vi "svl_Build dB Label (channel info).vi"(4 "width (-)":i16, 5 "number format":i16(ring) items=["Engineering", "Exponential", "Fractional", "Automatic"], 6 "include reference (T)":bool=TRUE, 7 "peak units":string, 8 "error in (no error)":errorcluster, 9 "precision (1)":i16=1, 10 "channel info":T1={"sensor sensitivity"=1000.0, "engineering units"=1, "dB reference"=1.0, "custom label"="EU", "weighting filter"=0, "pregain"=0.0} {"pregain" format="%.2f"; "weighting filter" items=["Linear", "A-weighting", "B-weighting", "C-weighting", "ITU-R 468-4", "Dolby", "CCITT", "C-message", "Wb", "Wc", "Wd", "We", "Wf", "Wh", "Wj", "Wk", "Wm", "AES17 20 kHz lowpass", "AES17 40 kHz lowpass", "AES17 20 kHz highpass", "AES17 40 kHz highpass"]; "dB reference" format="%^.1e"; "engineering units" items=["custom..."=0, "V"=1, "A"=21, "C"=30, "pC"=31, "s"=32, "-"=29, "Pa"=2, "N"=20, "g"=3, "m/s^2"=4, "m/s"=5, "m"=6, "mm/s"=12, "mm"=13, "micron/s"=14, "micron"=15, "in/s^2"=7, "in/s"=8, "in"=9, "mil/s"=10, "mil"=11, "rad/s^2"=16, "rad/s"=17, "rad"=18, "deg/s^2"=26, "deg/s"=27, "deg"=28, "RPM"=22, "cycle/s^2"=23, "Hz"=24, "cycle"=25, "strain"=19]; "sensor sensitivity" format="%#_5f"}, 11 "EU label":string) -> (0 "error out":errorcluster, 1 "dB reference [EU]":dbl format="%.2f", 2 "channel info":T1={"sensor sensitivity"=1000.0, "engineering units"=1, "dB reference"=1.0, "custom label"="EU", "weighting filter"=0, "pregain"=0.0} {"pregain" format="%.2f"; "weighting filter" items=["Linear", "A-weighting", "B-weighting", "C-weighting", "ITU-R 468-4", "Dolby", "CCITT", "C-message", "Wb", "Wc", "Wd", "We", "Wf", "Wh", "Wj", "Wk", "Wm", "AES17 20 kHz lowpass", "AES17 40 kHz lowpass", "AES17 20 kHz highpass", "AES17 40 kHz highpass"]; "dB reference" format="%^.1e"; "engineering units" items=["custom..."=0, "V"=1, "A"=21, "C"=30, "pC"=31, "s"=32, "-"=29, "Pa"=2, "N"=20, "g"=3, "m/s^2"=4, "m/s"=5, "m"=6, "mm/s"=12, "mm"=13, "micron/s"=14, "micron"=15, "in/s^2"=7, "in/s"=8, "in"=9, "mil/s"=10, "mil"=11, "rad/s^2"=16, "rad/s"=17, "rad"=18, "deg/s^2"=26, "deg/s"=27, "deg"=28, "RPM"=22, "cycle/s^2"=23, "Hz"=24, "cycle"=25, "strain"=19]; "sensor sensitivity" format="%#_5f"}, 3 "dB label":string)   [LabVIEW 2017]
uses:
  <vilib>/addons/_NISVFA/_Shared subVIs/Controls/svc_Channel Info.ctl
  <vilib>/addons/_NISVFA/_Shared subVIs/Controls/svc_Engineering Units Text Ring.ctl
  <vilib>/addons/_NISVFA/_Shared subVIs/Controls/svc_Weighting Filter Text Ring.ctl
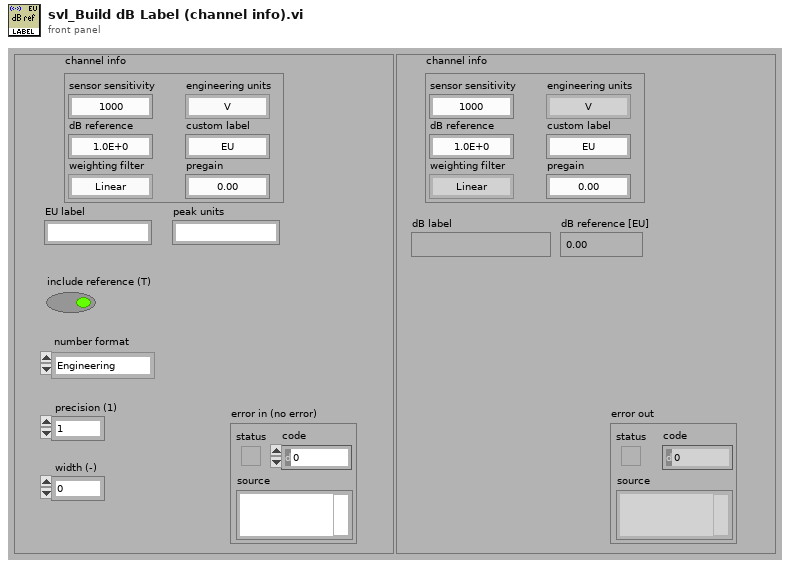
[diagram p1: front panel]
types:
  T1 = typedef "svc_Channel Info.ctl" = cluster{"sensor sensitivity":dbl, "engineering units":T2, "dB reference":dbl, "custom label":string, "weighting filter":T3, "pregain":dbl}
  T2 = typedef "svc_Engineering Units Text Ring.ctl" = u16
  T3 = typedef "svc_Weighting Filter Text Ring.ctl" = u16
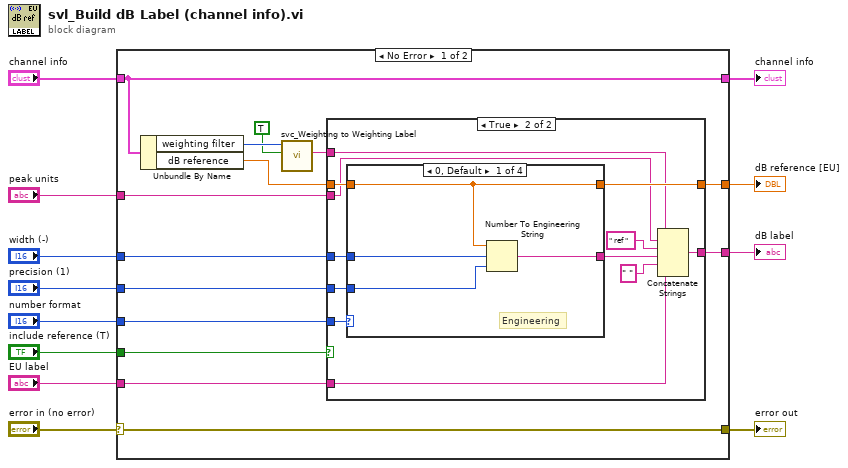
[diagram p0: block diagram]
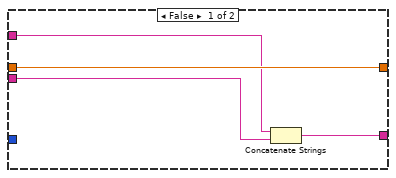
[diagram p2: hidden frame]
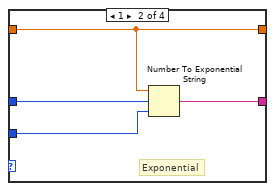
[diagram p3: hidden frame]
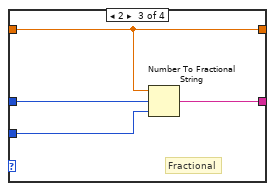
[diagram p4: hidden frame]
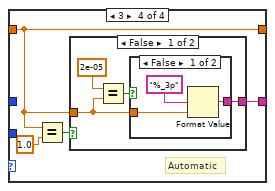
[diagram p5: hidden frame]
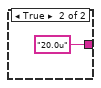
[diagram p6: hidden frame]
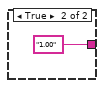
[diagram p7: hidden frame]
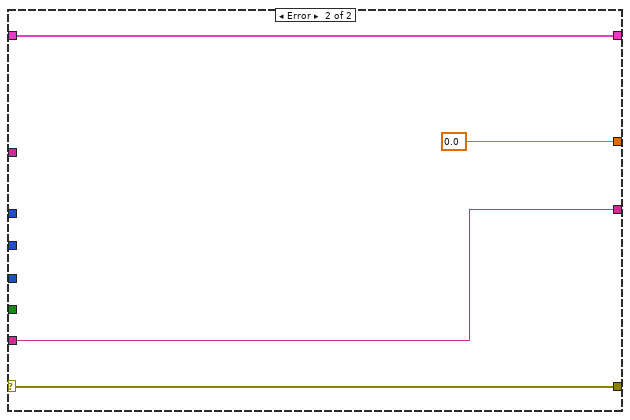
[diagram p8: hidden frame]
diagram:
  n1 = case shown="No Error" "error in (no error)" {
    selector: "error in (no error)" -> [w20 w71]
    tunnel: "include reference (T)" -> [w26 _]
    tunnel: "channel info" -> [w16 w70]
    tunnel: [w25 w69] -> w10
    tunnel: [w16 w70] -> w8
    tunnel: "EU label" -> [w22 w69]
    tunnel: "number format" -> [w21 _]
    tunnel: [w20 w71] -> w5
    tunnel: [w18 0.0 ("sensor sensitivity [mV/EU]")] -> w4
    tunnel: "precision (1)" -> [w15 _]
    tunnel: "width (-)" -> [w14 _]
    tunnel: "peak units" -> [w13 _]
    frame No Error {
      n2 = Unbundle By Name(w16) -> ("weighting filter"=w23:T3, "dB reference"=w19:dbl)
      n3 = call <vilib>:"svc_Weighting to Weighting Label.vi"("dB On (T)"=TRUE, "weighting filter"=w23) -> ("weighting string"=w24:string)  [unwired: 8 in, 1 out]
      n4 = case shown="True" w26 {
        tunnel: [w27 w41] -> w25
        tunnel: w24 -> [w28 w34]
        tunnel: w22 -> [_ w40]
        tunnel: w21 -> [_ w39]
        tunnel: w19 -> [w30 w38]
        tunnel: [w30 w37] -> w18
        tunnel: w15 -> [_ w33]
        tunnel: w14 -> [_ w32]
        tunnel: w13 -> [w29 w31]
        frame False {
          n5 = Concatenate Strings(w28, w29) -> (w27:string)
        }
        frame True {
          n6 = case shown="0, Default" w39 {
            tunnel: [w44 w50 w54 w58] -> w42
            tunnel: w32 -> [w45 w49 w53 _]
            tunnel: w33 -> [w46 w48 w52 _]
            tunnel: w38 -> [w43 w47 w51 w57]
            tunnel: [w43 w47 w51 w57] -> w37
            frame 0, Default {
              # "Engineering"
              n7 = Number To Engineering String(2:w46, 3:w45, 4:w43) -> (0:w44:string)  [unwired: 1 in]
            }
            frame 1 {
              # "Exponential"
              n8 = Number To Exponential String(number=w47, precision (6)=w48, 3:w49) -> (E-format string=w50:string)  [unwired: 1 in]
            }
            frame 2 {
              # "Fractional"
              n9 = Number To Fractional String(number=w51, width (-)=w53, precision (6)=w52) -> (F-format string=w54:string)  [unwired: 1 in]
            }
            frame 3 {
              # "Automatic"
              n10 = Equal?(x=w57, y=1.0) -> (x = y?=w55:bool)
              n11 = case shown="False" w55 {
                tunnel: [w62 "1.00" ("format string")] -> w58
                tunnel: w57 -> [w61 _]
                frame False {
                  n12 = Equal?(x=2e-05 ("y"), y=w61) -> (x = y?=w59:bool)
                  n13 = case shown="False" w59 {
                    tunnel: [w64 "20.0u" ("format string")] -> w62
                    tunnel: w61 -> [w63 _]
                    frame False {
                      n14 = Format Value(format string="%_3p", value (0)=w63) -> (output string=w64:string)  [unwired: 1 in]
                    }
                    frame True {
                    }
                  }
                }
                frame True {
                }
              }
            }
          }
          n15 = Concatenate Strings(w34, w31, " ref ", w42, " " ("custom label"), w40) -> (w41:string)
        }
      }
    }
    frame Error {
    }
  }
  "error out" <- w5
  "dB label" <- w10
  "dB reference [EU]" <- w4
  "channel info" <- w8
